vi "failUnlessGeneratedAndParsedOneToOne.vi"(4 "Convert EOL? (TRUE)":bool=TRUE, 6 "message (\"\")":string, 8 "error in":errorcluster, 9 "XML String":string, 10 "Data":variant, 11 "EasyXMLTest in":refnum<class "EasyXMLTest.lvclass">) -> (0 "error out":errorcluster, 1 "Produced Data":variant, 2 "Generated XML String":string, 3 "EasyXMLTest out":refnum<class "EasyXMLTest.lvclass">)   [LabVIEW 2013, in "EasyXMLTest.lvclass"]
doc: "This VI validates that the XML data generated is parsed back to the original data structure in a one-to-one fashion. It test both Flatten and Unflatten, in a single shot."
uses:
  EasyXMLTest.lvclass
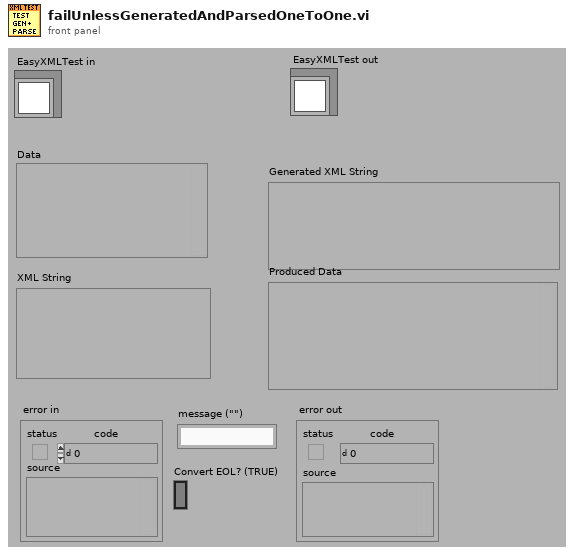
[diagram p1: front panel]
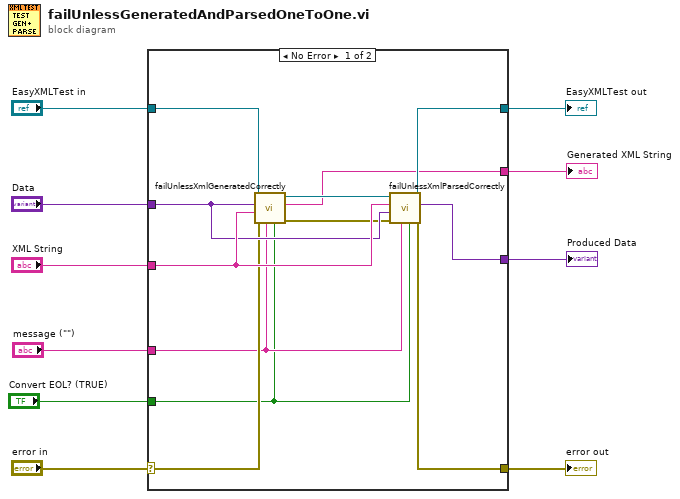
[diagram p0: block diagram]
diagram:
  n1 = case shown="No Error" "error in" {
    selector: "error in" -> [w15 w24]
    tunnel: "EasyXMLTest in" -> [w22 w23]
    tunnel: [w20 w23] -> w7
    tunnel: "XML String" -> [w19 _]
    tunnel: "Data" -> [w18 _]
    tunnel: [w16 w24] -> w10
    tunnel: "message (\"\")" -> [w14 _]
    tunnel: [w13 _] -> w3
    tunnel: [w12 _] -> w2
    tunnel: "Convert EOL? (TRUE)" -> [w11 _]
    frame No Error {
      n2 = call "failUnlessXmlGeneratedCorrectly.vi"("Convert EOL? (TRUE)"=w11, "message (\"\")"=w14, "error in"=w15, "expected XML string"=w19, "Input Data"=w18, "EasyXMLTest in"=w22) -> ("error out"=w17:errorcluster, "Generated XML String"=w13:string, "EasyXMLTest out"=w21:refnum<class "EasyXMLTest.lvclass">)  [unwired: 3 in]
      n3 = call "failUnlessXmlParsedCorrectly.vi"("Convert EOL? (TRUE)"=w11, "message (\"\")"=w14, "error in"=w17, "Expected Data"=w18, "XML String"=w19, "reference in"=w21) -> ("error out"=w16:errorcluster, "Produced Data"=w12:variant, "reference in"=w20:refnum<class "EasyXMLTest.lvclass">)  [unwired: 3 in]
    }
    frame Error {
    }
  }
  "error out" <- w10
  "EasyXMLTest out" <- w7
  "Generated XML String" <- w3
  "Produced Data" <- w2
